vi "Substract Strings.vi"(10 "format string 2":string, 11 "format string":string) -> (3 "substracted string":string)   [LabVIEW 2019, in "Day 8.lvlib"]
uses:
  Day 8.lvlib
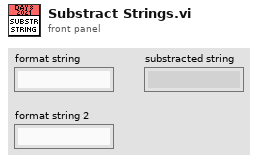
[diagram p1: front panel]
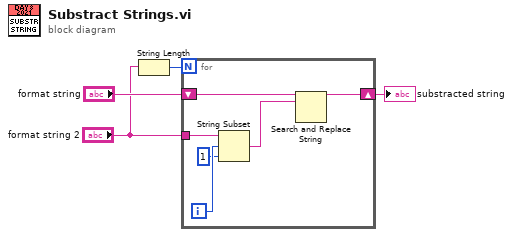
[diagram p0: block diagram]
diagram:
  n1 = String Length(string="format string 2") -> (length=w2:i32)
  n2 = for {
    N: w2 -> [_]
    tunnel: "format string 2" -> [w10]
    shift-right: [w7] -> w1
    shift-left: "format string" -> [w9]
    i -> [w6]
    n3 = String Subset(string=w10, offset (0)=w6, length (rest)=1 ("length (rest)")) -> (substring=w8:string)
    n4 = Search and Replace String(input string=w9, search string=w8) -> (result string=w7:string)  [unwired: 6 in, 3 out]
  }
  "substracted string" <- w1
